vi "Load Grid Save Synp AER.vi"() -> ()   [LabVIEW 2013]
uses:
  Synapses/Synapses.lvclass
  AER/AER.lvclass
  Cerebellum/Cerebellum.lvclass
panel:
  out "error out":errorcluster
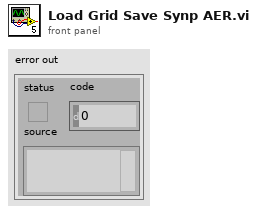
[diagram p1: front panel]
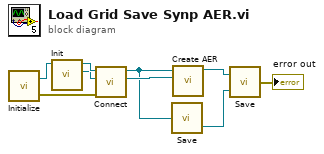
[diagram p0: block diagram]
diagram:
  n1 = call "Initialize.vi"() -> ("Grid out"=w5:refnum<class "Grid.lvclass">, "error out"=w8:errorcluster)  [unwired: 1 in]
  n2 = call "Init.vi"("Grid in"=w5) -> ("Grid out"=w7:refnum<class "Grid.lvclass">, "Synapses out"=w9:refnum<class "Synapses.lvclass">)  [unwired: 9 in]
  n3 = call "Connect.vi"(8:w8, "Grid in"=w7, "Synapses in"=w9) -> ("Grid out"=w6:refnum<class "Grid.lvclass">, "Synapses  out"=w2:refnum<class "Synapses.lvclass">)  [unwired: 7 in]
  n4 = call "Save.vi"("Synapses in"=w2) -> ("Synapses out"=w1:refnum<class "Synapses.lvclass">)  [unwired: 1 out]
  n5 = call "Create AER.vi"("Grid.lvclass"=w6, "Synapses in"=w2) -> ("AER.lvclass"=w4:refnum<class "AER.lvclass">)  [unwired: 6 in, 3 out]
  n6 = call "Save.vi"("Synapses in"=w1, "AER in"=w4) -> ("error out"=→"error out":errorcluster)
